vi "Main Tclk.vi"() -> ()   [LabVIEW 2018] (continued)
                      tunnel: w5362 -> [w5374] mode=indexing
                      tunnel: w5361 -> [w5373] mode=indexing
                      tunnel: [w5372] -> w5366 mode=indexing
                      tunnel: w5360 -> [w5371] mode=indexing
                      tunnel: w5359 -> [w5370] mode=indexing
                      tunnel: [w5369] -> w5365 mode=indexing
                      tunnel: u8 1 ("x") -> [w5368]
                      tunnel: [w5367] -> w5357 mode=indexing
                      n5995 = for {
                        tunnel: w5374 -> [w5381] mode=indexing
                        tunnel: w5373 -> [w5380] mode=indexing
                        tunnel: [w5379] -> w5372 mode=indexing
                        tunnel: w5371 -> [w5375] mode=indexing
                        tunnel: w5370 -> [w5378] mode=indexing
                        tunnel: [w5377] -> w5369 mode=indexing
                        tunnel: w5368 -> [w5376]
                        tunnel: [w5375] -> w5367 mode=indexing
                        n5996 = In Range and Coerce(upper limit=w5381, x=w5380, lower limit=w5376) -> (coerced(x)=w5379:u8)  [unwired: 1 out]
                        n5997 = In Range and Coerce(upper limit=w5375, x=w5378, lower limit=w5376) -> (coerced(x)=w5377:sgl)  [unwired: 1 out]
                      }
                    }
                    n5998 = Bundle By Name(cluster=w5358, "Primary X index"=w5366, "Y Grids"=w5357, "Primary Y index"=w5365) -> (w5364:T28)
                    n5999 = local write "Focus Index Options"(w5364) -> ()
                  }
                  frame True {
                    n6000 = for {
                      tunnel: w5384 -> [w5395] mode=indexing
                      tunnel: w5383 -> [w5394] mode=indexing
                      tunnel: [w5393] -> w5388 mode=indexing
                      tunnel: [w5392] -> w5387 mode=indexing
                      tunnel: [w5391] -> w5386 mode=indexing
                      tunnel: [w5390] -> w5385 mode=indexing
                      n6001 = for {
                        tunnel: w5395 -> [w5401] mode=indexing
                        tunnel: w5394 -> [w5400] mode=indexing
                        tunnel: [w5399] -> w5393 mode=indexing
                        tunnel: [w5398] -> w5392 mode=indexing
                        tunnel: [w5397] -> w5391 mode=indexing
                        tunnel: [w5396] -> w5390 mode=indexing
                        n6002 = To Single Precision Float(number=w5401) -> (single precision float=w5404:sgl)
                        n6003 = To Single Precision Float(number=w5400) -> (single precision float=w5403:sgl)
                        n6004 = expression code="x/2"(w5404) -> (w5405:sgl)
                        n6005 = expression code="x/2"(w5403) -> (w5402:sgl)
                        n6006 = Round Toward +Infinity(x=w5405) -> (ceil(x): smallest int >= x=w5398:sgl)
                        n6007 = Round Toward +Infinity(x=w5402) -> (ceil(x): smallest int >= x=w5396:sgl)
                        n6008 = expression code="x*2-1"(w5398) -> (w5399:sgl)
                        n6009 = expression code="x*2-1"(w5396) -> (w5397:sgl)
                      }
                    }
                    n6010 = Bundle By Name(cluster=w5382, "X Grids"=w5388, "Primary X index"=w5387, "Y Grids"=w5386, "Primary Y index"=w5385) -> (w5389:T28)
                    n6011 = local write "Focus Index Options"(w5389) -> ()
                  }
                }
              }
              frame Enabled {
              }
            }
            n6012 = local write "FI array for stop limit"(sgl[] [] ("FI array for stop limit")) -> ()
            n6013 = local read "Focus Index Options"() -> (w5335:T28)
            n6014 = local read "SEM Scan Parameters"() -> (w5336:T26)
            n6015 = call "Focus Grid Chooser.vi"("SEM Scan Parameters"=w5336, "Focus Index Options"=w5335) -> ("Focus Index Options Out"=w5337:T28)  [unwired: 9 in]
            n6016 = local write "Focus Index Options"(w5337) -> ()
          }
          event "Focus Index Options.Primary X index": Mouse Down; "Focus Index Options.Primary X index": Value Change {
            n6017 = event-data() -> ()  [unwired: 5 out]
            n6018 = disable-structure shown="Disabled" {
              frame Disabled {
                n6019 = local read "Focus Index Options"() -> (w5414:T28)
                n6020 = Unbundle By Name(w5414) -> ("Focus Index primary grid center"=w5419:bool, "X Grids"=w5418:u8[][], "Primary X index"=w5417:u8[][])
                n6021 = local read "SEM Scan Parameters"() -> (w5425:T26)
                n6022 = case shown="True" w5419 {
                  tunnel: w5418 -> [w5429 _]
                  tunnel: w5417 -> [_ w5435]
                  tunnel: [1.0 ("Data Entry Limits:Increment") 0.0 ("Data Entry Limits:Increment")] -> w5416
                  tunnel: [u8 1 ("x") w5433] -> w5412
                  tunnel: [w5428 w5434] -> w5411
                  tunnel: [T44."Enabled" ("Disabled") T44."Disabled and Grayed Out" ("Disabled")] -> w5410
                  frame False {
                    n6023 = Array Max & Min(array=w5429) -> (max value=w5428:u8)  [unwired: 3 out]
                  }
                  frame True {
                    n6024 = Array Max & Min(array=w5435) -> (max value=w5434:u8, min value=w5433:u8)  [unwired: 2 out]
                  }
                }
                n6025 = Unbundle By Name(w5414) -> ("Primary X index"=w5421:u8[][])
                n6026 = Unbundle By Name(w5425) -> ("X tiles"=w5424:u8, "Y tiles"=w5423:u8)
                n6027 = call "2D array edit.vi"("min"=w5412, "max"=w5411, "Set boundaries"=TRUE ("Set boundary"), "Disabled"=w5410, "Data Entry Limits:Increment"=w5416, "Display Format:Precision"=u8 0, "Rows"=w5423, "Columns"=w5424, "Caption.Text"="Primary X grid", "Input array"=w5421) -> ("Output array"=w5415:sgl[][])  [unwired: 1 in]
                n6028 = Bundle By Name(cluster=w5414, "Primary X index"=w5415) -> (w5413:T28)
                n6029 = local write "Focus Index Options"(w5413) -> ()
              }
              frame Enabled {
              }
            }
            n6030 = local write "FI array for stop limit"(sgl[] [] ("FI array for stop limit")) -> ()
            n6031 = local read "Focus Index Options"() -> (w5406:T28)
            n6032 = local read "SEM Scan Parameters"() -> (w5407:T26)
            n6033 = call "Focus Grid Chooser.vi"("SEM Scan Parameters"=w5407, "Focus Index Options"=w5406) -> ("Focus Index Options Out"=w5408:T28)  [unwired: 9 in]
            n6034 = local write "Focus Index Options"(w5408) -> ()
          }
          event "Focus Index Options.Primary Y index": Mouse Down; "Focus Index Options.Primary Y index": Value Change {
            n6035 = event-data() -> ()  [unwired: 5 out]
            n6036 = disable-structure shown="Disabled" {
              frame Disabled {
                n6037 = local read "Focus Index Options"() -> (w5445:T28)
                n6038 = Unbundle By Name(w5445) -> ("Focus Index primary grid center"=w5450:bool, "Y Grids"=w5449:u8[][], "Primary Y index"=w5448:u8[][])
                n6039 = local read "SEM Scan Parameters"() -> (w5456:T26)
                n6040 = case shown="False" w5450 {
                  tunnel: w5449 -> [w5460 _]
                  tunnel: w5448 -> [_ w5466]
                  tunnel: [1.0 ("Data Entry Limits:Increment") 0.0 ("Data Entry Limits:Increment")] -> w5447
                  tunnel: [u8 1 ("x") w5464] -> w5443
                  tunnel: [w5459 w5465] -> w5442
                  tunnel: [T44."Enabled" ("Disabled") T44."Disabled and Grayed Out" ("Disabled")] -> w5441
                  frame False {
                    n6041 = Array Max & Min(array=w5460) -> (max value=w5459:u8)  [unwired: 3 out]
                  }
                  frame True {
                    n6042 = Array Max & Min(array=w5466) -> (max value=w5465:u8, min value=w5464:u8)  [unwired: 2 out]
                  }
                }
                n6043 = Unbundle By Name(w5445) -> ("Primary Y index"=w5452:u8[][])
                n6044 = Unbundle By Name(w5456) -> ("X tiles"=w5455:u8, "Y tiles"=w5454:u8)
                n6045 = call "2D array edit.vi"("min"=w5443, "max"=w5442, "Set boundaries"=TRUE ("Set boundary"), "Disabled"=w5441, "Data Entry Limits:Increment"=w5447, "Display Format:Precision"=u8 0, "Rows"=w5454, "Columns"=w5455, "Caption.Text"="Primary Y grid", "Input array"=w5452) -> ("Output array"=w5446:sgl[][])  [unwired: 1 in]
                n6046 = Bundle By Name(cluster=w5445, "Primary Y index"=w5446) -> (w5444:T28)
                n6047 = local write "Focus Index Options"(w5444) -> ()
              }
              frame Enabled {
              }
            }
            n6048 = local write "FI array for stop limit"(sgl[] [] ("FI array for stop limit")) -> ()
            n6049 = local read "Focus Index Options"() -> (w5437:T28)
            n6050 = local read "SEM Scan Parameters"() -> (w5438:T26)
            n6051 = call "Focus Grid Chooser.vi"("SEM Scan Parameters"=w5438, "Focus Index Options"=w5437) -> ("Focus Index Options Out"=w5439:T28)  [unwired: 9 in]
            n6052 = local write "Focus Index Options"(w5439) -> ()
          }
          event "Det A": Mouse Down {
            n6053 = event-data() -> ("Button"=w5468:u16)  [unwired: 8 out]
            n6054 = case shown="1" w5468 {
              frame 0, Default {
              }
              frame 1 {
                n6055 = local read "Focus Index tiled"() -> (w5475:sgl[][])
                n6056 = local read "SEM Scan Parameters"() -> (w5472:T26)
                n6057 = Unbundle By Name(w5472) -> ("X tiles"=w5473:u8, "Y tiles"=w5474:u8)
                n6058 = call "2D array edit.vi"("Auto close (s)"=u32 15, "Display Format:Precision"=u8 3, "Rows"=w5474, "Columns"=w5473, "Caption.Text"="Focus Index", "Input array"=w5475) -> ()  [unwired: 5 in, 1 out]
              }
            }
          }
          event "Pre-reheat Y stig": Mouse Down {
            n6059 = event-data() -> ()  [unwired: 9 out]
            n6060 = local read "Pre-reheat Y stig"() -> (w5477:sgl[][])
            n6061 = local read "SEM Scan Parameters"() -> (w5481:T26)
            n6062 = Unbundle By Name(w5481) -> ("X tiles"=w5480:u8, "Y tiles"=w5479:u8)
            n6063 = call "2D array edit.vi"("Auto close (s)"=u32 15, "Display Format:Precision"=u8 2, "Rows"=w5479, "Columns"=w5480, "Caption.Text"="Pre-reheat Y stig (%)", "Input array"=w5477) -> ()  [unwired: 5 in, 1 out]
          }
          event "Align failed array": Mouse Down {
            n6064 = event-data() -> ()  [unwired: 9 out]
            n6065 = local read "Align failed array"() -> (w5484:bool[][])
            n6066 = call "2D boolean array show.vi"("Input array"=w5484, "Caption.Text"="Align failed", "Colors [4]"=cluster{u32, u32}[] [{5898240, 5898240}, {16711680, 16711680}, {1985280, 1985280}, {6618880, 6618880}] ("Colors [4] 3")) -> ()  [unwired: 8 in]
          }
          event "AF Success tiled": Mouse Down {
            n6067 = event-data() -> ()  [unwired: 9 out]
            n6068 = local read "AF Success tiled"() -> (w5487:bool[][])
            n6069 = call "2D boolean array show.vi"("Input array"=w5487, "Caption.Text"="Auto Focus Success", "Colors [4]"=cluster{u32, u32}[] [{1985280, 1985280}, {6618880, 6618880}, {1985280, 1985280}, {6618880, 6618880}]) -> ()  [unwired: 8 in]
          }
          event "ASX Success tiled": Mouse Down {
            n6070 = event-data() -> ()  [unwired: 9 out]
            n6071 = local read "ASX Success tiled"() -> (w5490:bool[][])
            n6072 = call "2D boolean array show.vi"("Input array"=w5490, "Caption.Text"="Auto Stig X Success", "Colors [4]"=cluster{u32, u32}[] [{1985280, 1985280}, {6618880, 6618880}, {1985280, 1985280}, {6618880, 6618880}]) -> ()  [unwired: 8 in]
          }
          event "ASY Success tiled": Mouse Down {
            n6073 = event-data() -> ()  [unwired: 9 out]
            n6074 = local read "ASY Success tiled"() -> (w5493:bool[][])
            n6075 = call "2D boolean array show.vi"("Input array"=w5493, "Caption.Text"="Auto Stig Y Success", "Colors [4]"=cluster{u32, u32}[] [{1985280, 1985280}, {6618880, 6618880}, {1985280, 1985280}, {6618880, 6618880}]) -> ()  [unwired: 8 in]
          }
          event "AAX Success tiled": Mouse Down {
            n6076 = event-data() -> ()  [unwired: 9 out]
            n6077 = local read "AAX Success tiled"() -> (w5496:bool[][])
            n6078 = call "2D boolean array show.vi"("Input array"=w5496, "Caption.Text"="Auto Align X Success", "Colors [4]"=cluster{u32, u32}[] [{1985280, 1985280}, {6618880, 6618880}, {1985280, 1985280}, {6618880, 6618880}]) -> ()  [unwired: 8 in]
          }
          event "AAY Success tiled": Mouse Down {
            n6079 = event-data() -> ()  [unwired: 9 out]
            n6080 = local read "AAY Success tiled"() -> (w5499:bool[][])
            n6081 = call "2D boolean array show.vi"("Input array"=w5499, "Caption.Text"="Auto Align Y Success", "Colors [4]"=cluster{u32, u32}[] [{1985280, 1985280}, {6618880, 6618880}, {1985280, 1985280}, {6618880, 6618880}]) -> ()  [unwired: 8 in]
          }
          event "Best WD (mm) tiled": Mouse Down {
            n6082 = event-data() -> ()  [unwired: 9 out]
            n6083 = local read "Best WD (mm) tiled"() -> (w5502:dbl[][])
            n6084 = local read "SEM Scan Parameters"() -> (w5506:T26)
            n6085 = Unbundle By Name(w5506) -> ("X tiles"=w5505:u8, "Y tiles"=w5504:u8)
            n6086 = call "2D array edit.vi"("Auto close (s)"=u32 15, "Display Format:Precision"=u8 4, "Rows"=w5504, "Columns"=w5505, "Caption.Text"="Best WD (mm)", "Input array"=w5502) -> ()  [unwired: 5 in, 1 out]
          }
          event "Best Stig X (%) tiled": Mouse Down {
            n6087 = event-data() -> ()  [unwired: 9 out]
            n6088 = local read "Best Stig X (%) tiled"() -> (w5509:dbl[][])
            n6089 = local read "SEM Scan Parameters"() -> (w5513:T26)
            n6090 = Unbundle By Name(w5513) -> ("X tiles"=w5512:u8, "Y tiles"=w5511:u8)
            n6091 = call "2D array edit.vi"("Auto close (s)"=u32 15, "Display Format:Precision"=u8 2, "Rows"=w5511, "Columns"=w5512, "Caption.Text"="Best Stig X (%)", "Input array"=w5509) -> ()  [unwired: 5 in, 1 out]
          }
          event "Best Stig Y (%) tiled": Mouse Down {
            n6092 = event-data() -> ()  [unwired: 9 out]
            n6093 = local read "Best Stig Y (%) tiled"() -> (w5516:dbl[][])
            n6094 = local read "SEM Scan Parameters"() -> (w5520:T26)
            n6095 = Unbundle By Name(w5520) -> ("X tiles"=w5519:u8, "Y tiles"=w5518:u8)
            n6096 = call "2D array edit.vi"("Auto close (s)"=u32 15, "Display Format:Precision"=u8 2, "Rows"=w5518, "Columns"=w5519, "Caption.Text"="Best Stig Y (%)", "Input array"=w5516) -> ()  [unwired: 5 in, 1 out]
          }
          event "Best Aln X (%) tiled": Mouse Down {
            n6097 = event-data() -> ()  [unwired: 9 out]
            n6098 = local read "Best Aln X (%) tiled"() -> (w5523:dbl[][])
            n6099 = local read "SEM Scan Parameters"() -> (w5527:T26)
            n6100 = Unbundle By Name(w5527) -> ("X tiles"=w5526:u8, "Y tiles"=w5525:u8)
            n6101 = call "2D array edit.vi"("Auto close (s)"=u32 15, "Display Format:Precision"=u8 2, "Rows"=w5525, "Columns"=w5526, "Caption.Text"="Best Align X (%)", "Input array"=w5523) -> ()  [unwired: 5 in, 1 out]
          }
          event "Best Aln Y (%) tiled": Mouse Down {
            n6102 = event-data() -> ()  [unwired: 9 out]
            n6103 = local read "Best Aln Y (%) tiled"() -> (w5530:dbl[][])
            n6104 = local read "SEM Scan Parameters"() -> (w5534:T26)
            n6105 = Unbundle By Name(w5534) -> ("X tiles"=w5533:u8, "Y tiles"=w5532:u8)
            n6106 = call "2D array edit.vi"("Auto close (s)"=u32 15, "Display Format:Precision"=u8 2, "Rows"=w5532, "Columns"=w5533, "Caption.Text"="Best Align Y (%)", "Input array"=w5530) -> ()  [unwired: 5 in, 1 out]
          }
          event "Auto Focus Graph": Mouse Down {
            n6107 = event-data() -> ("PlatMods"=w5546:T77)  [unwired: 8 out]
            n6108 = Unbundle By Name(w5546) -> ("Shift"=w5545:bool)
            n6109 = local read "AF Graph scales tiled"() -> (w5542:cluster{sgl, sgl, sgl, sgl}[][])
            n6110 = local read "Auto Focus Graph tiled"() -> (w5551:T4)
            n6111 = local read "AF Y tile"() -> (w5550:u8)
            n6112 = local read "AF X tile"() -> (w5549:u8)
            n6113 = local read "SEM Scan Parameters"() -> (w5548:T26)
            n6114 = Unbundle By Name(w5548) -> ("X tiles"=w5547:u8, "Y tiles"=w5544:u8)
            n6115 = case shown="True" w5545 {
              tunnel: w5551 -> [w5561 w5570]
              tunnel: w5550 -> [w5554 w5568]
              tunnel: w5549 -> [w5560 w5563]
              tunnel: w5547 -> [w5558 _]
              tunnel: w5544 -> [_ w5569]
              tunnel: [w5557 w5567] -> w5543
              tunnel: w5542 -> [w5556 w5566]
              tunnel: [w5555 w5565] -> w5541
              tunnel: [w5552 w5562] -> w5536
              frame False {
                n6116 = Increment(x=w5560) -> (x+1=w5559:u8)
                n6117 = Quotient & Remainder(x=w5559, y=w5558) -> (x-y*floor(x/y)=w5553:u8)  [unwired: 1 out]
                n6118 = Index Array(array=w5556, index (row)=w5554, index (col)=w5553) -> (element=w5555:cluster{sgl, sgl, sgl, sgl})
                n6119 = Index Array(array=w5561, index (dim 0)=w5554, index (dim 1)=w5553) -> (element=w5557:T75)  [unwired: 1 in]
                n6120 = local write "AF X tile"(w5553) -> ()
                n6121 = Build Array(w5554, w5553) -> (w5552:u8[])
              }
              frame True {
                n6122 = Increment(x=w5568) -> (x+1=w5571:u8)
                n6123 = Quotient & Remainder(x=w5571, y=w5569) -> (x-y*floor(x/y)=w5564:u8)  [unwired: 1 out]
                n6124 = Index Array(array=w5566, index (row)=w5564, index (col)=w5563) -> (element=w5565:cluster{sgl, sgl, sgl, sgl})
                n6125 = Index Array(array=w5570, index (dim 0)=w5564, index (dim 1)=w5563) -> (element=w5567:T75)  [unwired: 1 in]
                n6126 = local write "AF Y tile"(w5564) -> ()
                n6127 = Build Array(w5564, w5563) -> (w5562:u8[])
              }
            }
            n6128 = Unbundle(w5541) -> (w5540:sgl, w5539:sgl, w5538:sgl, w5537:sgl)
            n6129 = local write "Auto Focus Graph"(w5543) -> ()
            n6130 = property on="AF Success tiled" class="Arr (strict)"("Index Values"=w5536) -> ()  [unwired: 2 in, 2 out]
            n6131 = property on="Best WD (mm) tiled" class="Arr (strict)"("Index Values"=w5536) -> ()  [unwired: 2 in, 2 out]
            n6132 = property on="Best WD FI tiled" class="Arr (strict)"("Index Values"=w5536) -> ()  [unwired: 2 in, 2 out]
            n6133 = property on="Auto Focus Graph" class="XYGraph (strict)"("XScale.Maximum"=w5540, "XScale.Minimum"=w5539, "YScale.Maximum"=w5538, "YScale.Minimum"=w5537) -> ()  [unwired: 2 in, 2 out]
          }
          event "Auto Stig X": Mouse Down {
            n6134 = event-data() -> ("PlatMods"=w5582:T77)  [unwired: 8 out]
            n6135 = Unbundle By Name(w5582) -> ("Shift"=w5581:bool)
            n6136 = local read "ASX Graph scales tiled"() -> (w5578:cluster{sgl, sgl, sgl, sgl}[][])
            n6137 = local read "ASX Graph tiled"() -> (w5587:T4)
            n6138 = local read "ASX Y tile"() -> (w5586:u8)
            n6139 = local read "ASX X tile"() -> (w5585:u8)
            n6140 = local read "SEM Scan Parameters"() -> (w5584:T26)
            n6141 = Unbundle By Name(w5584) -> ("X tiles"=w5583:u8, "Y tiles"=w5580:u8)
            n6142 = case shown="False" w5581 {
              tunnel: w5587 -> [w5597 w5606]
              tunnel: w5586 -> [w5590 w5604]
              tunnel: w5585 -> [w5596 w5599]
              tunnel: w5583 -> [w5594 _]
              tunnel: w5580 -> [_ w5605]
              tunnel: [w5593 w5603] -> w5579
              tunnel: w5578 -> [w5592 w5602]
              tunnel: [w5591 w5601] -> w5577
              tunnel: [w5588 w5598] -> w5572
              frame False {
                n6143 = Increment(x=w5596) -> (x+1=w5595:u8)
                n6144 = Quotient & Remainder(x=w5595, y=w5594) -> (x-y*floor(x/y)=w5589:u8)  [unwired: 1 out]
                n6145 = Index Array(array=w5592, index (row)=w5590, index (col)=w5589) -> (element=w5591:cluster{sgl, sgl, sgl, sgl})
                n6146 = Index Array(array=w5597, index (dim 0)=w5590, index (dim 1)=w5589) -> (element=w5593:T75)  [unwired: 1 in]
                n6147 = local write "ASX X tile"(w5589) -> ()
                n6148 = Build Array(w5590, w5589) -> (w5588:u8[])
              }
              frame True {
                n6149 = Increment(x=w5604) -> (x+1=w5607:u8)
                n6150 = Quotient & Remainder(x=w5607, y=w5605) -> (x-y*floor(x/y)=w5600:u8)  [unwired: 1 out]
                n6151 = Index Array(array=w5602, index (row)=w5600, index (col)=w5599) -> (element=w5601:cluster{sgl, sgl, sgl, sgl})
                n6152 = Index Array(array=w5606, index (dim 0)=w5600, index (dim 1)=w5599) -> (element=w5603:T75)  [unwired: 1 in]
                n6153 = local write "ASX Y tile"(w5600) -> ()
                n6154 = Build Array(w5600, w5599) -> (w5598:u8[])
              }
            }
            n6155 = Unbundle(w5577) -> (w5576:sgl, w5575:sgl, w5574:sgl, w5573:sgl)
            n6156 = local write "Auto Stig X"(w5579) -> ()
            n6157 = property on="ASX Success tiled" class="Arr (strict)"("Index Values"=w5572) -> ()  [unwired: 2 in, 2 out]
            n6158 = property on="Best Stig X (%) tiled" class="Arr (strict)"("Index Values"=w5572) -> ()  [unwired: 2 in, 2 out]
            n6159 = property on="Best Stig X FI tiled" class="Arr (strict)"("Index Values"=w5572) -> ()  [unwired: 2 in, 2 out]
            n6160 = property on="Auto Stig X" class="XYGraph (strict)"("XScale.Maximum"=w5576, "XScale.Minimum"=w5575, "YScale.Maximum"=w5574, "YScale.Minimum"=w5573) -> ()  [unwired: 2 in, 2 out]
          }
          event "Auto Stig Y": Mouse Down {
            n6161 = event-data() -> ("PlatMods"=w5618:T77)  [unwired: 8 out]
            n6162 = Unbundle By Name(w5618) -> ("Shift"=w5617:bool)
            n6163 = local read "ASY Graph scales tiled"() -> (w5614:cluster{sgl, sgl, sgl, sgl}[][])
            n6164 = local read "ASY Graph tiled"() -> (w5623:T4)
            n6165 = local read "ASY Y tile"() -> (w5622:u8)
            n6166 = local read "ASY X tile"() -> (w5621:u8)
            n6167 = local read "SEM Scan Parameters"() -> (w5620:T26)
            n6168 = Unbundle By Name(w5620) -> ("X tiles"=w5619:u8, "Y tiles"=w5616:u8)
            n6169 = case shown="True" w5617 {
              tunnel: w5623 -> [w5633 w5642]
              tunnel: w5622 -> [w5626 w5640]
              tunnel: w5621 -> [w5632 w5635]
              tunnel: w5619 -> [w5630 _]
              tunnel: w5616 -> [_ w5641]
              tunnel: [w5629 w5639] -> w5615
              tunnel: w5614 -> [w5628 w5638]
              tunnel: [w5627 w5637] -> w5613
              tunnel: [w5624 w5634] -> w5608
              frame False {
                n6170 = Increment(x=w5632) -> (x+1=w5631:u8)
                n6171 = Quotient & Remainder(x=w5631, y=w5630) -> (x-y*floor(x/y)=w5625:u8)  [unwired: 1 out]
                n6172 = Index Array(array=w5628, index (row)=w5626, index (col)=w5625) -> (element=w5627:cluster{sgl, sgl, sgl, sgl})
                n6173 = Index Array(array=w5633, index (dim 0)=w5626, index (dim 1)=w5625) -> (element=w5629:T75)  [unwired: 1 in]
                n6174 = local write "ASY X tile"(w5625) -> ()
                n6175 = Build Array(w5626, w5625) -> (w5624:u8[])
              }
              frame True {
                n6176 = Increment(x=w5640) -> (x+1=w5643:u8)
                n6177 = Quotient & Remainder(x=w5643, y=w5641) -> (x-y*floor(x/y)=w5636:u8)  [unwired: 1 out]
                n6178 = Index Array(array=w5638, index (row)=w5636, index (col)=w5635) -> (element=w5637:cluster{sgl, sgl, sgl, sgl})
                n6179 = Index Array(array=w5642, index (dim 0)=w5636, index (dim 1)=w5635) -> (element=w5639:T75)  [unwired: 1 in]
                n6180 = local write "ASY Y tile"(w5636) -> ()
                n6181 = Build Array(w5636, w5635) -> (w5634:u8[])
              }
            }
            n6182 = Unbundle(w5613) -> (w5612:sgl, w5611:sgl, w5610:sgl, w5609:sgl)
            n6183 = local write "Auto Stig Y"(w5615) -> ()
            n6184 = property on="ASY Success tiled" class="Arr (strict)"("Index Values"=w5608) -> ()  [unwired: 2 in, 2 out]
            n6185 = property on="Best Stig Y (%) tiled" class="Arr (strict)"("Index Values"=w5608) -> ()  [unwired: 2 in, 2 out]
            n6186 = property on="Best Stig Y FI tiled" class="Arr (strict)"("Index Values"=w5608) -> ()  [unwired: 2 in, 2 out]
            n6187 = property on="Auto Stig Y" class="XYGraph (strict)"("XScale.Maximum"=w5612, "XScale.Minimum"=w5611, "YScale.Maximum"=w5610, "YScale.Minimum"=w5609) -> ()  [unwired: 2 in, 2 out]
          }
          event "Auto Aln X": Mouse Down {
            n6188 = event-data() -> ("PlatMods"=w5654:T77)  [unwired: 8 out]
            n6189 = Unbundle By Name(w5654) -> ("Shift"=w5653:bool)
            n6190 = local read "AAX Graph scales tiled"() -> (w5650:cluster{sgl, sgl, sgl, sgl}[][])
            n6191 = local read "AAX Graph tiled"() -> (w5659:T4)
            n6192 = local read "AAX Y tile"() -> (w5658:u8)
            n6193 = local read "AAX X tile"() -> (w5657:u8)
            n6194 = local read "SEM Scan Parameters"() -> (w5656:T26)
            n6195 = Unbundle By Name(w5656) -> ("X tiles"=w5655:u8, "Y tiles"=w5652:u8)
            n6196 = case shown="False" w5653 {
              tunnel: w5659 -> [w5669 w5678]
              tunnel: w5658 -> [w5662 w5676]
              tunnel: w5657 -> [w5668 w5671]
              tunnel: w5655 -> [w5666 _]
              tunnel: w5652 -> [_ w5677]
              tunnel: [w5665 w5675] -> w5651
              tunnel: w5650 -> [w5664 w5674]
              tunnel: [w5663 w5673] -> w5649
              tunnel: [w5660 w5670] -> w5644
              frame False {
                n6197 = Increment(x=w5668) -> (x+1=w5667:u8)
                n6198 = Quotient & Remainder(x=w5667, y=w5666) -> (x-y*floor(x/y)=w5661:u8)  [unwired: 1 out]
                n6199 = local write "AAX X tile"(w5661) -> ()
                n6200 = Index Array(array=w5664, index (row)=w5662, index (col)=w5661) -> (element=w5663:cluster{sgl, sgl, sgl, sgl})
                n6201 = Index Array(array=w5669, index (dim 0)=w5662, index (dim 1)=w5661) -> (element=w5665:T75)  [unwired: 1 in]
                n6202 = Build Array(w5662, w5661) -> (w5660:u8[])
              }
              frame True {
                n6203 = Increment(x=w5676) -> (x+1=w5679:u8)
                n6204 = Quotient & Remainder(x=w5679, y=w5677) -> (x-y*floor(x/y)=w5672:u8)  [unwired: 1 out]
                n6205 = local write "AAX Y tile"(w5672) -> ()
                n6206 = Index Array(array=w5674, index (row)=w5672, index (col)=w5671) -> (element=w5673:cluster{sgl, sgl, sgl, sgl})
                n6207 = Index Array(array=w5678, index (dim 0)=w5672, index (dim 1)=w5671) -> (element=w5675:T75)  [unwired: 1 in]
                n6208 = Build Array(w5672, w5671) -> (w5670:u8[])
              }
            }
            n6209 = Unbundle(w5649) -> (w5648:sgl, w5647:sgl, w5646:sgl, w5645:sgl)
            n6210 = property on="AAX Success tiled" class="Arr (strict)"("Index Values"=w5644) -> ()  [unwired: 2 in, 2 out]
            n6211 = property on="Best Aln X (%) tiled" class="Arr (strict)"("Index Values"=w5644) -> ()  [unwired: 2 in, 2 out]
            n6212 = property on="Best Aln X FI tiled" class="Arr (strict)"("Index Values"=w5644) -> ()  [unwired: 2 in, 2 out]
            n6213 = local write "Auto Aln X"(w5651) -> ()
            n6214 = property on="Auto Aln X" class="XYGraph (strict)"("XScale.Maximum"=w5648, "XScale.Minimum"=w5647, "YScale.Maximum"=w5646, "YScale.Minimum"=w5645) -> ()  [unwired: 2 in, 2 out]
          }
          event "Auto Aln Y": Mouse Down {
            n6215 = event-data() -> ("PlatMods"=w5690:T77)  [unwired: 8 out]
            n6216 = Unbundle By Name(w5690) -> ("Shift"=w5689:bool)
            n6217 = local read "AAY Graph scales tiled"() -> (w5686:cluster{sgl, sgl, sgl, sgl}[][])
            n6218 = local read "AAY Graph tiled"() -> (w5695:T4)
            n6219 = local read "AAY Y tile"() -> (w5694:u8)
            n6220 = local read "AAY X tile"() -> (w5693:u8)
            n6221 = local read "SEM Scan Parameters"() -> (w5692:T26)
            n6222 = Unbundle By Name(w5692) -> ("X tiles"=w5691:u8, "Y tiles"=w5688:u8)
            n6223 = case shown="True" w5689 {
              tunnel: w5695 -> [w5705 w5714]
              tunnel: w5694 -> [w5698 w5712]
              tunnel: w5693 -> [w5704 w5707]
              tunnel: w5691 -> [w5702 _]
              tunnel: w5688 -> [_ w5713]
              tunnel: [w5701 w5711] -> w5687
              tunnel: w5686 -> [w5700 w5710]
              tunnel: [w5699 w5709] -> w5685
              tunnel: [w5696 w5706] -> w5680
              frame False {
                n6224 = Increment(x=w5704) -> (x+1=w5703:u8)
                n6225 = Quotient & Remainder(x=w5703, y=w5702) -> (x-y*floor(x/y)=w5697:u8)  [unwired: 1 out]
                n6226 = local write "AAY X tile"(w5697) -> ()
                n6227 = Index Array(array=w5700, index (row)=w5698, index (col)=w5697) -> (element=w5699:cluster{sgl, sgl, sgl, sgl})
                n6228 = Index Array(array=w5705, index (dim 0)=w5698, index (dim 1)=w5697) -> (element=w5701:T75)  [unwired: 1 in]
                n6229 = Build Array(w5698, w5697) -> (w5696:u8[])
              }
              frame True {
                n6230 = Increment(x=w5712) -> (x+1=w5715:u8)
                n6231 = Quotient & Remainder(x=w5715, y=w5713) -> (x-y*floor(x/y)=w5708:u8)  [unwired: 1 out]
                n6232 = local write "AAY Y tile"(w5708) -> ()
                n6233 = Index Array(array=w5710, index (row)=w5708, index (col)=w5707) -> (element=w5709:cluster{sgl, sgl, sgl, sgl})
                n6234 = Index Array(array=w5714, index (dim 0)=w5708, index (dim 1)=w5707) -> (element=w5711:T75)  [unwired: 1 in]
                n6235 = Build Array(w5708, w5707) -> (w5706:u8[])
              }
            }
            n6236 = Unbundle(w5685) -> (w5684:sgl, w5683:sgl, w5682:sgl, w5681:sgl)
            n6237 = property on="AAY Success tiled" class="Arr (strict)"("Index Values"=w5680) -> ()  [unwired: 2 in, 2 out]
            n6238 = property on="Best Aln Y (%) tiled" class="Arr (strict)"("Index Values"=w5680) -> ()  [unwired: 2 in, 2 out]
            n6239 = property on="Best Aln Y FI tiled" class="Arr (strict)"("Index Values"=w5680) -> ()  [unwired: 2 in, 2 out]
            n6240 = local write "Auto Aln Y"(w5687) -> ()
            n6241 = property on="Auto Aln Y" class="XYGraph (strict)"("XScale.Maximum"=w5684, "XScale.Minimum"=w5683, "YScale.Maximum"=w5682, "YScale.Minimum"=w5681) -> ()  [unwired: 2 in, 2 out]
          }
        }
        n6242 = Unbundle By Name(w3154) -> ("status"=w3152:bool)
        n6243 = Or(x=w3152, y=w3151) -> (x .or. y?=w3153:bool)
      }
      n6244 = while {
        stop <- w889 stop-if-true
        n6245 = Wait Until Next ms Multiple(millisecond multiple=u32 100) -> ()  [unwired: 1 out]
        n6246 = case shown="True" "Start Reheat" {
          frame False {
          }
          frame True {
            n6247 = stacked-sequence {
              frame #0 {
                n6248 = local read "Milling para"() -> (w894:T35)
                n6249 = local read "Auto reheat running"() -> (w892:bool)
                n6250 = Unbundle By Name(w894) -> ("Auto Profile"=w893:bool)
                n6251 = And(x=w893, y=w892) -> (x .and. y?=w891:bool)
                n6252 = case shown="True" w891 {
                  frame False {
                  }
                  frame True {
                    n6253 = stacked-sequence {
                      frame #0 {
                        n6254 = local write "FIB Profile"(TRUE ("FIB Profile")) -> ()
                        n6255 = local write "Enable logging"(FALSE ("Enable logging")) -> ()
                        n6256 = local read "Hardware Configuration"() -> (w902:T25)
                        n6257 = Unbundle By Name(w902) -> ("Shutter Drive"=w901:tag)
                        n6258 = local read "Damping"() -> (w895:bool)
                        n6259 = call "Shutter Swing V3.vi"("Shutter Drive"=w901, "Damping"=w895, "Shutter close"=TRUE) -> ("Shutter close fdbk"=w900:bool, "Fail #"=w896:u8, "SEM shutter status"=w897:string)  [unwired: 2 in, 4 out]
                        n6260 = Greater Than 0?(x=w896) -> (x > 0?=w899:bool)
                        n6261 = local write "SEM Shutter"(w900) -> ()
                        n6262 = local write "SEM shutter status"(w897) -> ()
                        n6263 = local write "Fail #"(w896) -> ()
                        n6264 = local write "SEM shutter failed active"(w899) -> ()
                      }
                      frame #1 {
                        n6265 = Wait (ms)(milliseconds to wait=u32 2000) -> ()  [unwired: 1 out]
                      }
                      frame #2 {
                        n6266 = local read "Machine Type"() -> (w906:u8)
                        n6267 = case shown="2" w906 {
                          frame 0, Default {
                            w908 = sgl 90.0 ("UL-Ang")
                            n6268 = local read "HV Data Output"() -> (w924:T18)
                            n6269 = local read "Active logging channels"() -> (w912:string)
                            n6270 = local read "FIB HW Config"() -> (w915:T23)
                            n6271 = local read "FIB Options"() -> (w914:T33)
                            n6272 = local read "Milling para"() -> (w918:T35)
                            n6273 = local read "FIB profile X center (um)"() -> (w923:dbl)
                            n6274 = local read "FIB profile Y center (um)"() -> (w922:dbl)
                            n6275 = local read "FIB Scan Parameters"() -> (w917:T32)
                            n6276 = local read "Parameter Names"() -> (w911:string[])
                            n6277 = Bundle By Name(cluster=w917, "Frame line rampdown ratio"=0.0, "Oversampling"=u16 5) -> (w913:T32)
                            n6278 = Bundle By Name(cluster=w918, "X size (um)"=sgl 0.1, "Z size (um)"=sgl 10.0 ("Y size (um)"), "X center (um)"=w923, "Z center (um)"=w922, "UL-Ang"=w908, "UR-Ang"=w908) -> (w919:T35)
                            n6279 = local read "Api"() -> (w907:refnum<k7>)
                            n6280 = call "FIB profile.vi"("ActiveX Container"=w907, "HV Data Output"=w924, "Parameter Names"=w911, "Active logging channels"=w912, "Scan Para"=w913, "Milling para"=w919, "Options"=w914, "HW Config"=w915) -> ("Measurements"=w910:dbl[][])  [unwired: 1 in, 2 out]
                            n6281 = local write "Measurements"(w910) -> ()
                          }
                          frame 2 {
                            w926 = sgl 90.0 ("UL-Ang")
                            n6282 = local read "Active logging channels"() -> (w931:string)
                            n6283 = local read "FIB HW Config"() -> (w934:T23)
                            n6284 = local read "FIB Options"() -> (w933:T33)
                            n6285 = local read "Milling para"() -> (w937:T35)
                            n6286 = local read "FIB profile X center (um)"() -> (w942:dbl)
                            n6287 = local read "FIB profile Y center (um)"() -> (w941:dbl)
                            n6288 = local read "FIB Scan Parameters"() -> (w936:T32)
                            n6289 = local read "Parameter Names"() -> (w930:string[])
                            n6290 = local read "Capella HV Data Output"() -> (w927:T17)
                            n6291 = Bundle By Name(cluster=w936, "Frame line rampdown ratio"=0.0, "Oversampling"=u16 5) -> (w932:T32)
                            n6292 = Bundle By Name(cluster=w937, "X size (um)"=sgl 0.1, "Z size (um)"=sgl 10.0 ("Y size (um)"), "X center (um)"=w942, "Z center (um)"=w941, "UL-Ang"=w926, "UR-Ang"=w926) -> (w938:T35)
                            n6293 = local read "Api"() -> (w925:refnum<k7>)
                            n6294 = call "FIB profile.vi"("ActiveX Container"=w925, "Capella HV Data Output"=w927, "Parameter Names"=w930, "Active logging channels"=w931, "Scan Para"=w932, "Milling para"=w938, "Options"=w933, "HW Config"=w934) -> ("Measurements"=w929:dbl[][])  [unwired: 1 in, 2 out]
                            n6295 = local write "Measurements"(w929) -> ()
                          }
                        }
                      }
                      frame #3 {
                        n6296 = local write "FIB Profile"(FALSE ("FIB Profile")) -> ()
                        n6297 = local write "Enable logging"(TRUE ("Enable logging")) -> ()
                      }
                    }
                  }
                }
              }
              frame #1 {
                n6298 = local read "Machine Type"() -> (w945:u8)
                n6299 = case shown="2" w945 {
                  selector: w945 -> [w946 _ w1037]
                  frame 0, Default {
                    n6300 = stacked-sequence {
                      tunnel: w946 -> [_ _ _ _ _ _ _ _ w1031]
                      frame #0 {
                        n6301 = local read "Reheat start file"() -> (w947:path)
                        n6302 = File/Directory Info(path=w947) -> (path out=w950:path, error out=w948:errorcluster)  [unwired: 1 in, 5 out]
                        n6303 = Unbundle By Name(w948) -> ("status"=w949:bool)
                        n6304 = case shown="False" w949 {
                          tunnel: w950 -> [w951 _]
                          frame False {
                            n6305 = Delete(path (use dialog)=w951) -> ()  [unwired: 4 in, 3 out]
                          }
                          frame True {
                          }
                        }
                      }
                      frame #1 {
                        n6306 = local read "Reheat complete file"() -> (w954:path)
                        n6307 = local read "Reheat stopped file"() -> (w953:path)
                        n6308 = local write "Reheat completed"(FALSE ("Reheat completed")) -> ()
                        n6309 = local write "Status Tabs"(T11."FIB" ("Status Tabs")) -> ()
                        n6310 = File/Directory Info(path=w954) -> (path out=w960:path, last mod=w956:timestamp, error out=w962:errorcluster)  [unwired: 1 in, 4 out]
                        n6311 = File/Directory Info(path=w953) -> (path out=w959:path, error out=w957:errorcluster)  [unwired: 1 in, 5 out]
                        n6312 = Unbundle By Name(w962) -> ("status"=w961:bool)
                        n6313 = Unbundle By Name(w957) -> ("status"=w958:bool)
                        n6314 = case shown="False" w961 {
                          tunnel: w960 -> [w965 _]
                          tunnel: w956 -> [w964 _]
                          frame False {
                            n6315 = Delete(path (use dialog)=w965) -> ()  [unwired: 4 in, 3 out]
                            "Last auto reheat" <- w964
                          }
                          frame True {
                          }
                        }
                        n6316 = case shown="False" w958 {
                          tunnel: w959 -> [w963 _]
                          frame False {
                            n6317 = Delete(path (use dialog)=w963) -> ()  [unwired: 4 in, 3 out]
                          }
                          frame True {
                          }
                        }
                      }
                      frame #2 {
                        n6318 = local read "Auto reheat running"() -> (w973:bool)
                        n6319 = Get Date/Time In Seconds() -> (seconds since 1Jan1904=w970:timestamp)
                        "Reheat time" <- w970
                        n6320 = local read "Last auto reheat"() -> (w969:timestamp)
                        n6321 = local read "Turn FIB Gun on"() -> (w966:bool)
                        n6322 = property on="Request to stop reheat" class="Bool (strict)"("DisabledEnum"=T44."Enabled" ("Disabled")) -> ()  [unwired: 2 in, 2 out]
                        n6323 = Subtract(x=w970, y=w969) -> (x-y=w977:dbl)
                        n6324 = expression code="x/60"(w977) -> (w976:dbl)
                        n6325 = Less Or Equal?(x=w976, y=120.0) -> (x <= y?=w974:bool)
                        n6326 = And(x=w973, y=w974) -> (x .and. y?=w968:bool)
                        n6327 = Or(x=w968, y=w966) -> (x .or. y?=w967:bool)
                        n6328 = case shown="True" w967 {
                          tunnel: "Reheat Parameters" -> [w979 w985]
                          tunnel: [w979 w981] -> w971
                          frame False {
                          }
                          frame True {
                            n6329 = Bundle By Name(cluster=w985, "Filament I (A)"=sgl 0.1, "Reheat time (s)"=sgl 1.0, "Calculate V/I slope"=FALSE, "Disable Reheat Retries"=TRUE) -> (w981:T1)
                          }
                        }
                        "Actual Reheat Parameters" <- w971
                      }
                      frame #3 {
                        n6330 = local read "Actual Reheat Parameters"() -> (w987:T1)
                        n6331 = call "Write FIB reheat file.vi"("Reheat Parameters"=w987) -> ()  [unwired: 11 in]
                        "Send reheat start email" <- TRUE
                      }
                      frame #4 {
                        n6332 = while {
                          stop <- w1003 stop-if-true
                          n6333 = local read "Reheat complete file"() -> (w999:path)
                          n6334 = local read "Reheat stopped file"() -> (w1000:path)
                          n6335 = Wait Until Next ms Multiple(millisecond multiple=u32 100) -> ()  [unwired: 1 out]
                          n6336 = File/Directory Info(path=w999) -> (path out=w995:path, error out=w994:errorcluster)  [unwired: 1 in, 5 out]
                          n6337 = File/Directory Info(path=w1000) -> (path out=w996:path, error out=w997:errorcluster)  [unwired: 1 in, 5 out]
                          n6338 = local read "Stop"() -> (w1004:bool)
                          n6339 = Unbundle By Name(w994) -> ("status"=w993:bool)
                          n6340 = Unbundle By Name(w997) -> ("status"=w998:bool)
                          n6341 = Not(x=w993) -> (.not. x?=w1001:bool)
                          n6342 = Not(x=w998) -> (.not. x?=w1002:bool)
                          n6343 = case shown="True" w1001 {
                            selector: w1001 -> [w1011 w1012]
                            tunnel: w995 -> [_ w1013]
                            tunnel: [w1011 w1012] -> w990
                            frame False {
                            }
                            frame True {
                              "Reheat log file" <- w1013
                            }
                          }
                          n6344 = case shown="True" w1002 {
                            selector: w1002 -> [w1008 w1009]
                            tunnel: w996 -> [_ w1010]
                            tunnel: [w1008 w1009] -> w989
                            frame False {
                            }
                            frame True {
                              n6345 = local write "Reheat log file"(w1010) -> ()
                            }
                          }
                          n6346 = Or(x=w990, y=w989) -> (x .or. y?=w992:bool)
                          n6347 = Or(x=w992, y=w1004) -> (x .or. y?=w1003:bool)
                          n6348 = case shown="True" "Stop Reheat" {
                            frame False {
                              n6349 = local write "Status message"("FIB reheat in progress..." ("Status message")) -> ()
                            }
                            frame True {
                              n6350 = local write "Status message"("Stopping FIB reheat" ("Status message")) -> ()
                              n6351 = call "Write FIB reheat file.vi"("Start"=FALSE) -> ()  [unwired: 11 in]
                            }
                          }
                        }
                      }
                      frame #5 {
                        n6352 = Wait (ms)(milliseconds to wait=u32 500) -> ()  [unwired: 1 out]
                      }
                      frame #6 {
                        w1021 = u8 1 items=["HV Data", "Reheat"] ("Log file type")
                        n6353 = local read "Reheat log file"() -> (w1023:path)
                        n6354 = call "Read FIB Log Files.vi"("Log file type"=w1021, "Log file path"=w1023) -> ("Reheat Output"=→"Reheat Output":T21)  [unwired: 8 in, 1 out]
                        n6355 = call "Read FIB Log Files.vi"("Log file path"=path "C:/Program Files (x86)/FEI Company/BDS/LogHVData.log") -> ("HV Data Output"=w1016:T118)  [unwired: 9 in, 1 out]
                        n6356 = File/Directory Info(path=path "C:/Program Files (x86)/FEI Company/BDS/Reheat/Stop.txt" ("Log file path")) -> (path out=w1020:path, error out=w1018:errorcluster)  [unwired: 1 in, 5 out]
                        n6357 = local write "HV Data Output"(w1016) -> ()
                        n6358 = Unbundle By Name(w1018) -> ("status"=w1019:bool)
                        n6359 = case shown="False" w1019 {
                          tunnel: w1020 -> [w1024 _]
                          frame False {
                            n6360 = Delete(path (use dialog)=w1024) -> ()  [unwired: 4 in, 3 out]
                          }
                          frame True {
                          }
                        }
                      }
                      frame #7 {
                        n6361 = local read "Stop Reheat"() -> (w1027:bool)
                        n6362 = local read "Reheat Output"() -> (w1026:T21)
                        n6363 = Unbundle By Name(w1026) -> ("Reheat Success"=w1025:bool)
                        n6364 = Select(t="Reheat Stopped" ("Status message"), s=w1027, f="Reheat Completed" ("Status message")) -> (s? t:f=w1030:string)
                        n6365 = local write "Status message"(w1030) -> ()
                        n6366 = local write "Start FIB HV DataLog"(w1025) -> ()
                      }
                      frame #8 {
                        n6367 = local read "Reheat Output"() -> (w1034:T21)
                        n6368 = local read "FIB Reheat Log Files"() -> (w1033:path)
                        n6369 = local read "Reheat time"() -> (w1032:timestamp)
                        n6370 = local read "HV Data Output"() -> (w1036:T18)
                        n6371 = local read "Actual Reheat Parameters"() -> (w1035:T1)
                        n6372 = call "Write FIB reheat log.vi"("HV Data Output"=w1036, "Reheat Output"=w1034, "Reheat Parameters"=w1035, "Reheat time"=w1032, "Machine Type"=w1031, "Log file path"=w1033) -> ()  [unwired: 6 in]
                      }
                    }
                  }
                  frame 1 {
                  }
                  frame 2 {
                    n6373 = stacked-sequence {
                      tunnel: w1037 -> [_ _ _ _ _ _ w1155]
                      frame #0 {
                        n6374 = local read "Api"() -> (w1040:refnum<k7>)
                        n6375 = local write "Status Tabs"(T11."FIB" ("Status Tabs")) -> ()
                        n6376 = local write "Reheat completed"(FALSE ("Reheat completed")) -> ()
                        n6377 = property on="Request to stop reheat" class="Bool (strict)"("DisabledEnum"=T44."Enabled" ("Disabled")) -> ()  [unwired: 2 in, 2 out]
                        n6378 = call "SmartSEM Remote API set float.vi"("vValue"=sgl 1.0, "lpszParam"="DP_FIB_BLANKED", "ActiveX Container"=w1040) -> ("error out"=w1038:errorcluster, "reference out"=w1039:refnum<k7>)  [unwired: 7 in]
                        n6379 = call "SmartSEM Remote API get FIB HV data.vi"("error in"=w1038, "ActiveX Container"=w1039) -> ("Capella HV Data Output"=w1043:T17)  [unwired: 6 in, 3 out]
                        n6380 = local write "Capella HV Data Output"(w1043) -> ()
                      }
                      frame #1 {
                        n6381 = Get Date/Time In Seconds() -> (seconds since 1Jan1904=w1047:timestamp)
                        n6382 = local read "Api"() -> (w1050:refnum<k7>)
                        n6383 = local write "Send reheat start email"(TRUE) -> ()
                        n6384 = local write "Reheat time"(w1047) -> ()
